vi "Simple Get File.vi"(0 "remote file uri":string, 1 "username":string, 2 "password":string, 7 "local file path":path, 11 "error in (no error)":errorcluster) -> (8 "local file path out":path, 15 "error out":errorcluster)   [LabVIEW 2020, in "NI_WebDAV.lvlib"]
doc: "Returns a file or multiple files or the raw binary contents of a file or multiple files from a remote WebDAV server or target. You must manually select the polymorphic instance you want to use."
uses:
  <vilib>/WebDAVClient/NI_WebDAV.lvlib
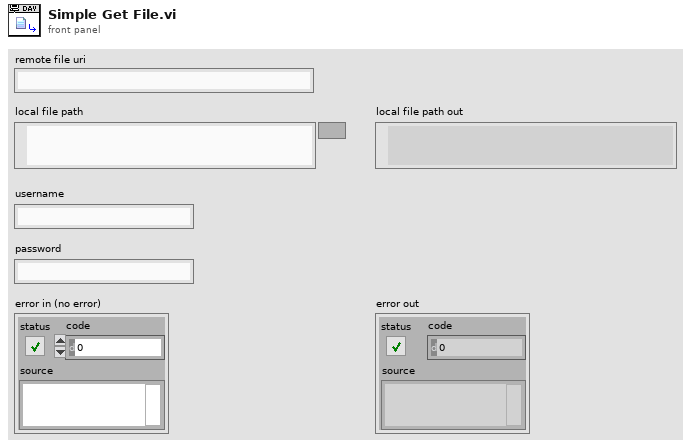
[diagram p1: front panel]
types:
  T1 = typedef "NI_WebDAV.lvlib/SessionHandle.ctl" = refnum<k1>
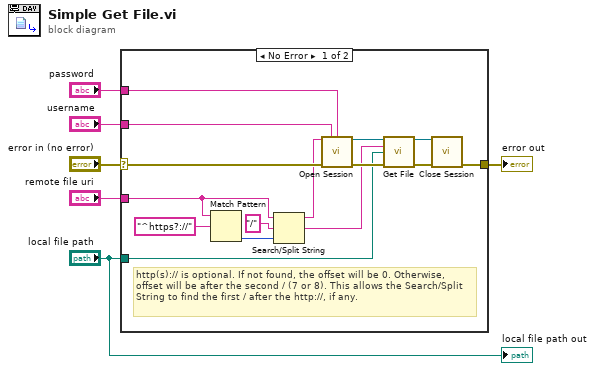
[diagram p0: block diagram]
diagram:
  n1 = case shown="No Error" "error in (no error)" {
    selector: "error in (no error)" -> [w21 w22]
    tunnel: "remote file uri" -> [w7 _]
    tunnel: "username" -> [w20 _]
    tunnel: "password" -> [w19 _]
    tunnel: "local file path" -> [w16 _]
    tunnel: [w13 w22] -> w1
    frame No Error {
      # "http(s):// is optional. If not found, the offset will be 0. Otherwise, offset will be after the second / (7 or 8). This allows the Search/Split String to find the first / after the http://, if any."
      n2 = Match Pattern(string=w7, regular expression="^https?://") -> (offset past match=w12:i32)  [unwired: 1 in, 3 out]
      n3 = Search/Split String(string=w7, search string/char (-)="/", offset (0)=w12) -> (substring before match=w8:string, match + rest of string=w9:string)  [unwired: 1 out]
      n4 = call <vilib>:"Open Session.vi"("host uri prefix"=w8, "username"=w20, "password"=w19, "error in (no error)"=w21) -> ("session handle out"=w17:T1, "error out"=w18:errorcluster)  [unwired: 10 in]
      n5 = call <vilib>:"Get File.vi"("session handle"=w17, "relative uri"=w9, "local file path"=w16, "error in (no error)"=w18) -> ("session handle out"=w14:T1, "error out"=w15:errorcluster)  [unwired: 9 in, 1 out]
      n6 = call <vilib>:"Close Session.vi"("session handle"=w14, "error in (no error)"=w15) -> ("error out"=w13:errorcluster)  [unwired: 13 in]
    }
    frame Error {
    }
  }
  "error out" <- w1
  "local file path out" <- "local file path"
